vi "Dimmer BaseStation With UI.vi"() -> ()   [LabVIEW 2014, in "ESP8266 WiFi Wrapper.lvlib"]
uses:
  <vilib>/Aledyne-TSXperts/Arduino Compatible Compiler for LabVIEW/addons/ESP8266 WiFi Wrapper/ESP8266 WiFi Wrapper.lvlib
  <vilib>/Aledyne-TSXperts/Arduino Compatible Compiler for LabVIEW/Arduino Compatible Compiler for LabVIEW.lvlib
panel:
  in  "DNS address":u8[](array[numeric])=[1, 2, 3, 4]
  in  "IP address":u8[](array[numeric])=[192, 168, 0, 42]
  in  "Gateway":u8[](array[numeric])=[192, 168, 0, 1]
  in  "Subnet mask":u8[](array[numeric])=[255, 255, 255, 0]
  in  "Password":string="12345678"
  in  "SSID":string="ESP8266 Wifi Example"
  in  "Listen Port":u8=80
  in  "error in (no error)":errorcluster
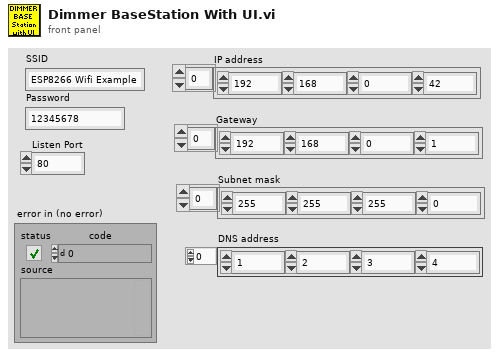
[diagram p1: front panel]
types:
  T1 = enum16{"WIFI_OFF", "WIFI_STA", "WIFI_AP", "WIFI_AP_STA"}
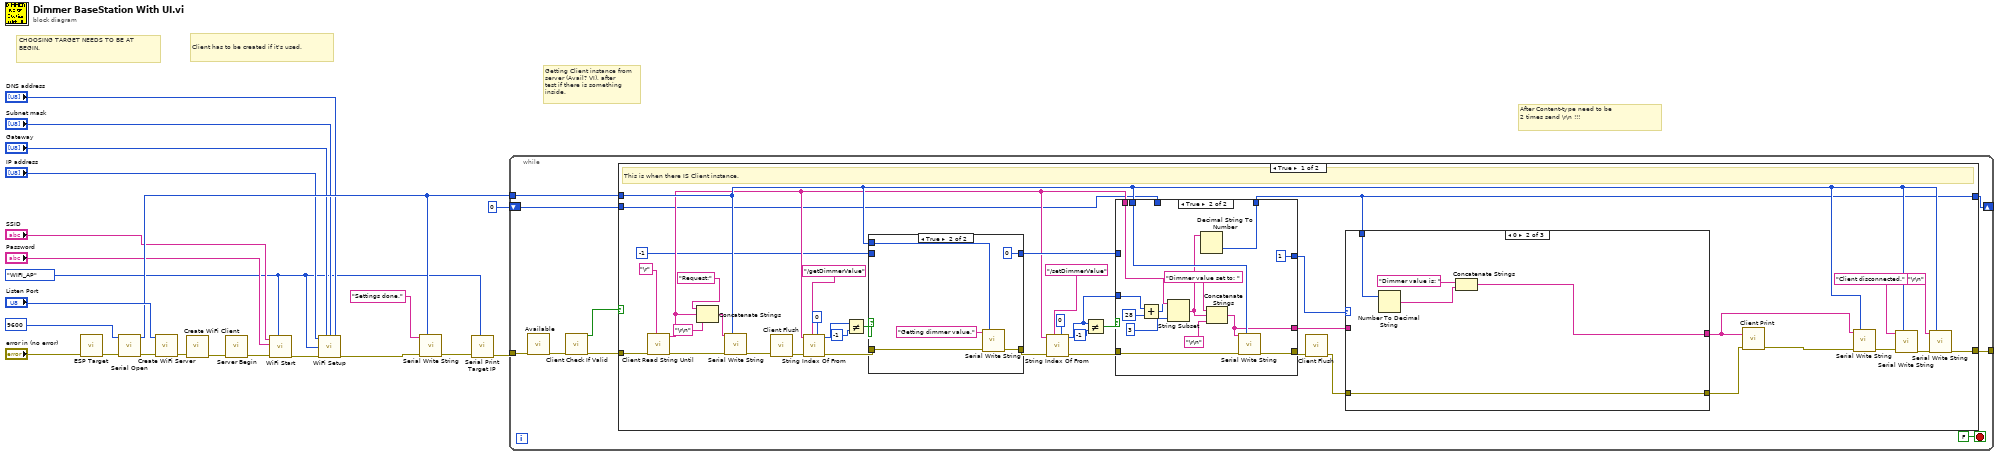
[diagram p0: block diagram]
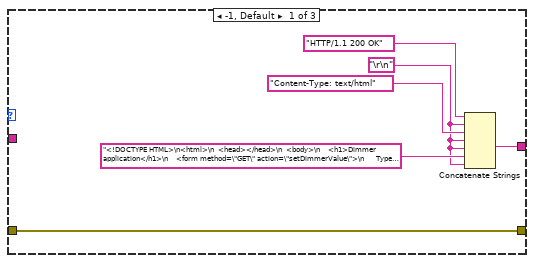
[diagram p2: hidden frame]
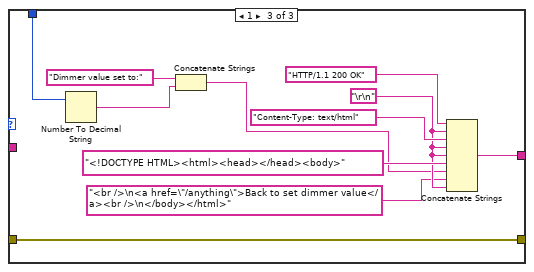
[diagram p3: hidden frame]
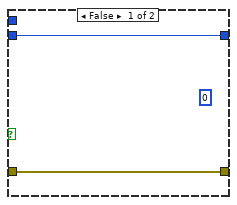
[diagram p5: hidden frame]
diagram:
  w2 = T1."WIFI_AP" ("WiFi Server Mode")
  # "After Content-type need to be\n2 times send \\r\\n !!!"
  # "Getting Client instance from\nserver (Avail? VI), after\ntest if there is something\ninside."
  # "CHOOSING TARGET NEEDS TO BE AT BEGIN."
  # "Client has to be created if it's used."
  n1 = call <vilib>:"ESP Target.vi"("Error In"="error in (no error)") -> ("Error Out"=w18:errorcluster)  [unwired: 10 in]
  n2 = call <vilib>:"Serial Open.vi"("Speed"=u32 9600, "error in (no error)"=w18) -> ("Instance"=w16:u8, "error out"=w21:errorcluster)  [unwired: 12 in]
  n3 = call <vilib>:"Create WiFi Server.vi"("Error In"=w21, "Listen Port"="Listen Port") -> ("Error Out"=w19:errorcluster)  [unwired: 9 in]
  n4 = call <vilib>:"Create WiFi Client.vi"("Error In"=w19) -> ("Error Out"=w12:errorcluster)  [unwired: 10 in]
  n5 = call <vilib>:"Server Begin.vi"("Error In"=w12) -> ("Error Out"=w14:errorcluster)  [unwired: 10 in]
  n6 = call <vilib>:"WiFi Start.vi"("WiFi Mode"=w2, "Error In"=w14, "Password"="Password", "SSID"="SSID") -> ("Error Out"=w13:errorcluster)  [unwired: 7 in]
  n7 = call <vilib>:"WiFi Setup.vi"("IP address"="IP address", "Gateway address"="Gateway", "Subnet mask"="Subnet mask", "DNS address"="DNS address", "WiFi Mode"=w2, "Error In"=w13) -> ("Error Out"=w11:errorcluster)  [unwired: 9 in]
  n8 = call <vilib>:"Serial Write String.vi"("String"="Settings done.", "Instance"=w16, "error in (no error)"=w11) -> ("error out"=w4:errorcluster)  [unwired: 12 in]
  n9 = call <vilib>:"Serial Print Target IP.vi"("WiFi Mode"=w2, "Error In"=w4) -> ("Error Out"=w3:errorcluster)  [unwired: 9 in]
  n10 = while {
    tunnel: [w29] -> _
    tunnel: w16 -> [w28]
    tunnel: w3 -> [w25]
    shift-right: [w24] -> _
    shift-left: u8 0 ("Start from") -> [w23]
    stop <- FALSE stop-if-true
    n11 = call <vilib>:"Available.vi"("Error In"=w25) -> ("Error Out"=w26:errorcluster)  [unwired: 10 in]
    n12 = call <vilib>:"Client Check If Valid.vi"("Error In"=w26) -> ("Error Out"=w27:errorcluster, "Is Null?"=w30:bool)  [unwired: 9 in]
    n13 = case shown="True" w30 {
      tunnel: w27 -> [w70 w118]
      tunnel: [w58 w118] -> w29
      tunnel: w28 -> [w44 _]
      tunnel: w23 -> [w33 w117]
      tunnel: [w32 w117] -> w24
      frame True {
        # "This is when there IS Client instance."
        n14 = call <vilib>:"Client Read String Until.vi"("Terminator char"="\r" ("Carriage Return Constant"), "Error In"=w70) -> ("Error Out"=w63:errorcluster, "Read String"=w40:string)  [unwired: 8 in]
        n15 = Concatenate Strings("Request:" ("string"), w40, "\r\n" ("End of Line Constant")) -> (w57:string)
        n16 = call <vilib>:"Serial Write String.vi"("String"=w57, "Instance"=w44, "error in (no error)"=w63) -> ("error out"=w62:errorcluster)  [unwired: 12 in]
        n17 = call <vilib>:"Client Flush.vi"("Error In"=w62) -> ("Error Out"=w50:errorcluster)  [unwired: 10 in]
        n18 = call <vilib>:"String Index Of From.vi"("Start from"=u8 0, "Find string"="/getDimmerValue" ("IndexOf String"), "Error In"=w50, "Input String"=w40) -> ("Error Out"=w49:errorcluster, "index"=w35:i8)  [unwired: 6 in]
        n19 = Not Equal?(x=w35, y=i8 -1) -> (x != y?=w68:bool)
        n20 = case shown="True" w68 {
          tunnel: [w111 w116] -> w47
          tunnel: w49 -> [w111 w115]
          tunnel: w44 -> [_ w114]
          tunnel: i8 -1 ("Start from") -> [w110 _]
          tunnel: [w110 i8 0 ("Start from")] -> w41
          frame False {
            (unwired) i8 0 ("index")
          }
          frame True {
            n21 = call <vilib>:"Serial Write String.vi"("String"="Getting dimmer value.", "Instance"=w114, "error in (no error)"=w115) -> ("error out"=w116:errorcluster)  [unwired: 12 in]
          }
        }
        n22 = call <vilib>:"String Index Of From.vi"("Start from"=u8 0, "Find string"="/setDimmerValue" ("IndexOf String"), "Error In"=w47, "Input String"=w40) -> ("Error Out"=w46:errorcluster, "index"=w43:i8)  [unwired: 6 in]
        n23 = Not Equal?(x=w43, y=i8 -1) -> (x != y?=w65:bool)
        n24 = case shown="True" w65 {
          tunnel: [w95 w109] -> w64
          tunnel: w46 -> [w95 w107]
          tunnel: w44 -> [_ w108]
          tunnel: w43 -> [_ w104]
          tunnel: [w94 i8 1 ("Start from")] -> w37
          tunnel: w41 -> [w94 _]
          tunnel: w40 -> [_ w105]
          tunnel: [_ w100] -> w36
          tunnel: w33 -> [w93 _]
          tunnel: [w93 w96] -> w32
          frame False {
          }
          frame True {
            n25 = Add(x=w104, y=i8 28) -> (x+y=w99:i8)
            n26 = String Subset(string=w105, offset (0)=w99, length (rest)=3 ("length (rest)")) -> (substring=w97:string)
            n27 = Decimal String To Number(string=w97) -> (number=w96:i32)  [unwired: 2 in, 1 out]
            n28 = Concatenate Strings("Dimmer value set to: " ("IndexOf String"), w97, "\r\n" ("End of Line Constant")) -> (w100:string)
            n29 = call <vilib>:"Serial Write String.vi"("String"=w100, "Instance"=w108, "error in (no error)"=w107) -> ("error out"=w109:errorcluster)  [unwired: 12 in]
          }
        }
        n30 = call <vilib>:"Client Flush.vi"("Error In"=w64) -> ("Error Out"=w39:errorcluster)  [unwired: 10 in]
        n31 = case shown="0" w37 {
          tunnel: [w72 w77 w83] -> w53
          tunnel: w39 -> [w76 w81 w92]
          tunnel: [w76 w81 w92] -> w38
          tunnel: w36 -> [_ _ _]
          tunnel: w32 -> [_ w79 w82]
          frame -1, Default {
            w71 = "\r\n" ("End of Line Constant")
            n32 = Concatenate Strings("HTTP/1.1 200 OK", w71, "Content-Type: text/html", w71, w71, "<!DOCTYPE HTML>\n<html>\n  <head></head>\n  <body>\n    <h1>Dimmer application</h1>\n    <form method=\"GET\" action=\"setDimmerValue\">\n      Type value (0-255)<input type=\"number\" name=\"dimmerValue\" value=0 \\><br \\>\n      <input type=\"submit\" value=\"Send\" \\>\n    </form>\n  </body>\n</html>", w71) -> (w72:string)
          }
          frame 0 {
            n33 = Number To Decimal String(number=w79) -> (decimal integer string=w78:string)  [unwired: 1 in]
            n34 = Concatenate Strings("Dimmer value is: " ("string"), w78) -> (w77:string)
          }
          frame 1 {
            w88 = "\r\n" ("End of Line Constant")
            n35 = Number To Decimal String(number=w82) -> (decimal integer string=w84:string)  [unwired: 1 in]
            n36 = Concatenate Strings("Dimmer value set to:" ("string"), w84) -> (w85:string)
            n37 = Concatenate Strings("HTTP/1.1 200 OK", w88, "Content-Type: text/html", w88, w88, "<!DOCTYPE HTML><html><head></head><body>", w85, "<br />\n<a href=\"/anything\">Back to set dimmer value</a><br />\n</body></html>" ("string"), w88) -> (w83:string)
          }
        }
        n38 = call <vilib>:"Client Print.vi"("Error In"=w38, "Input String"=w53) -> ("Error Out"=w52:errorcluster)  [unwired: 9 in]
        n39 = call <vilib>:"Serial Write String.vi"("String"=w53, "Instance"=w44, "error in (no error)"=w52) -> ("error out"=w54:errorcluster)  [unwired: 12 in]
        n40 = call <vilib>:"Serial Write String.vi"("String"="Client disconnected.", "Instance"=w44, "error in (no error)"=w54) -> ("error out"=w61:errorcluster)  [unwired: 12 in]
        n41 = call <vilib>:"Serial Write String.vi"("String"="\r\n" ("End of Line Constant"), "Instance"=w44, "error in (no error)"=w61) -> ("error out"=w58:errorcluster)  [unwired: 12 in]
      }
      frame False {
        # "No Client instance, do nothing."
      }
    }
  }
